vi "Turn to Angle.vi"(9 "Current Angle":dbl(slide) scale=-1080.0..1080.0, 10 "Angle to Get":dbl(slide) scale=-1080.0..1080.0) -> (1 "New Angle to Get":dbl(slide) scale=-1080.0..1080.0)   [LabVIEW 2019]
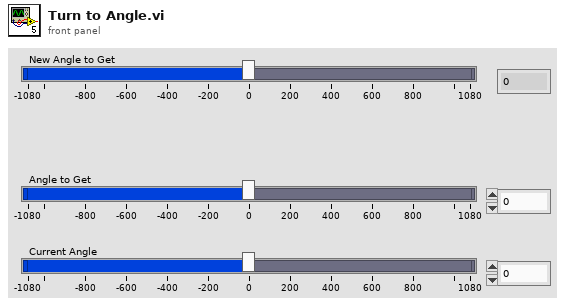
[diagram p1: front panel]
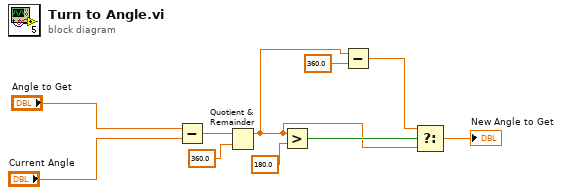
[diagram p0: block diagram]
diagram:
  n1 = Subtract(x="Angle to Get", y="Current Angle") -> (x-y=w8:dbl)
  n2 = Quotient & Remainder(x=w8, y=360.0) -> (x-y*floor(x/y)=w1:dbl)  [unwired: 1 out]
  n3 = Greater?(x=w1, y=180.0) -> (0:w2:bool)
  n4 = Subtract(x=w1, y=360.0) -> (x-y=w4:dbl)
  n5 = Select(t=w4, s=w2, f=w1) -> (s? t:f=→"New Angle to Get":dbl)
